vi "例4-14.vi"() -> ()   [LabVIEW 2019]
panel:
  out "输出数组":dbl[][](array[numeric])
  in  "输入数组":dbl[](array[numeric])
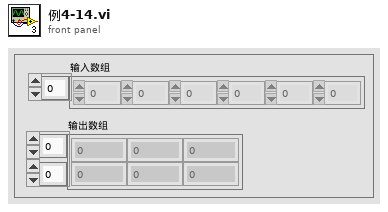
[diagram p1: front panel]
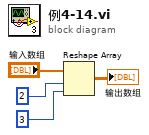
[diagram p0: block diagram]
diagram:
  n1 = Reshape Array("输入数组", 2, 3) -> (→"输出数组":dbl[][])
